vi "TurnDistance.vi"(7 "Timeout":dbl, 8 "Error In":errorcluster, 9 "Initation?":bool, 10 "MaxSpeed":dbl, 11 "Degrees":dbl) -> (0 "Error Out":errorcluster, 2 "Succesful":bool, 3 "Finished":bool)   [LabVIEW 2020]
uses:
  <vilib>/Utility/semaphor.llb/Obtain Semaphore Reference.vi
  <vilib>/Rock Robotics/WPI/ThirdParty/JAS_Junk/TrajLib/Timer_Reset.vi
  DriveGlobals.vi
  <vilib>/Rock Robotics/WPI/ThirdParty/JAS_Junk/TrajLib/Trajectory_Library.lvlib
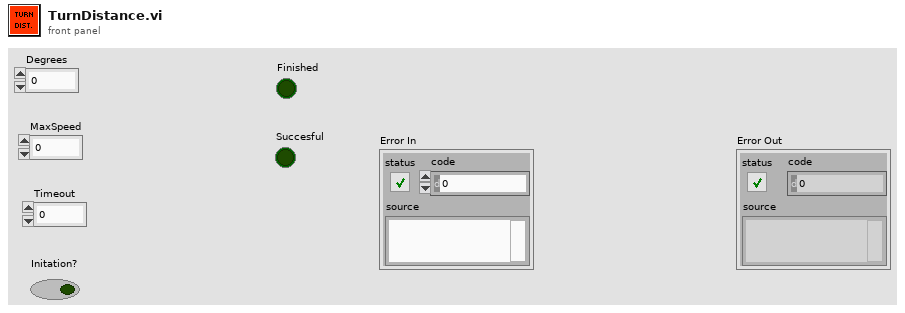
[diagram p1: front panel]
types:
  T1 = typedef "Trajectory_Library.lvlib/TIMER.ctl" = cluster{"StartTime":dbl, "Accumulated TIme":dbl, "Running":bool, "semaphore":T2}
  T2 = typedef "Semaphore RefNum" = refnum<k1>
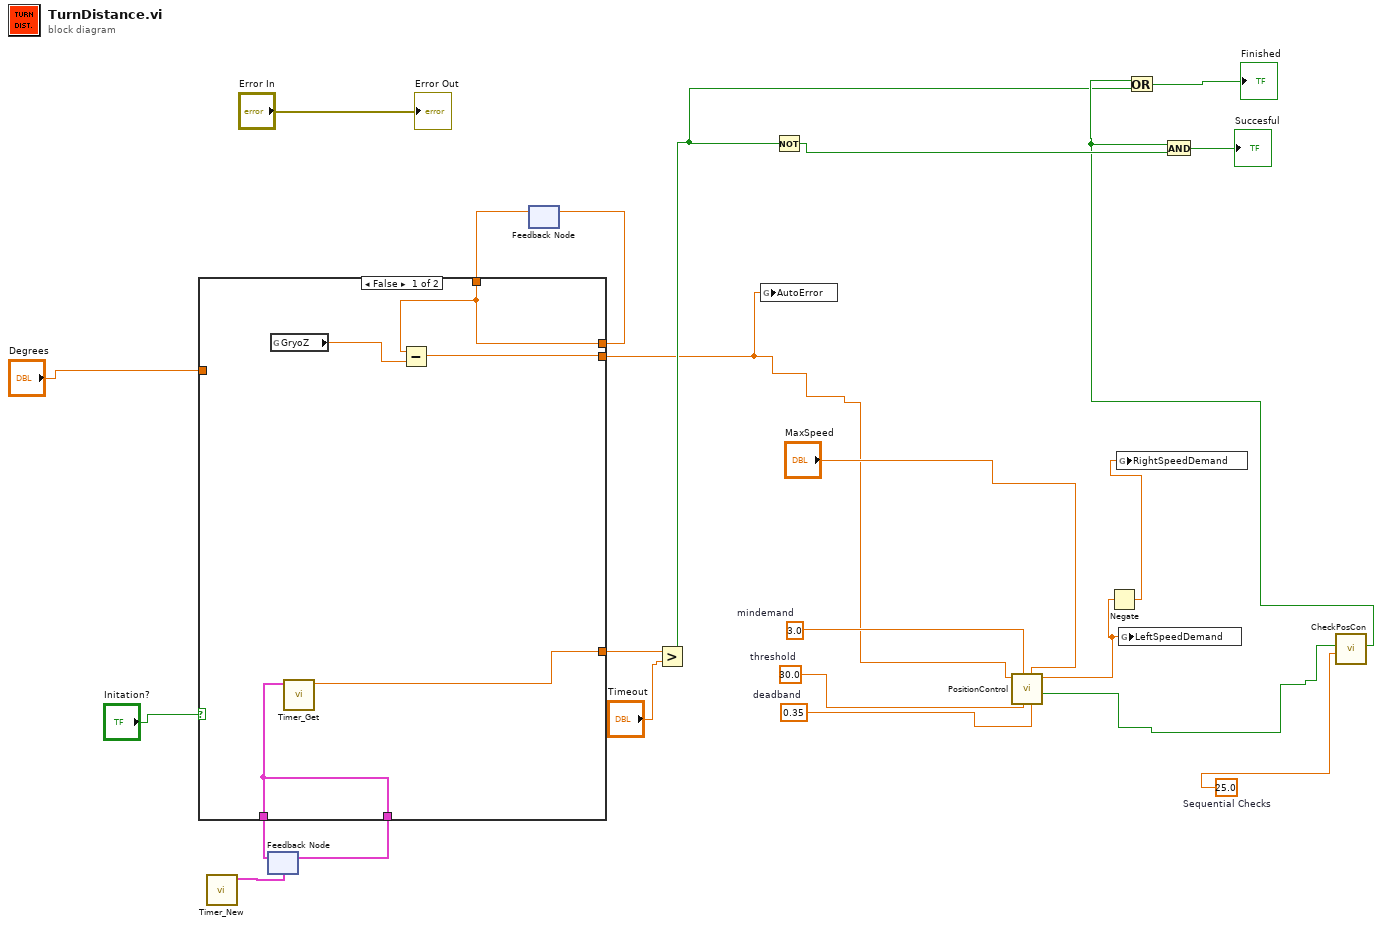
[diagram p0: block diagram]
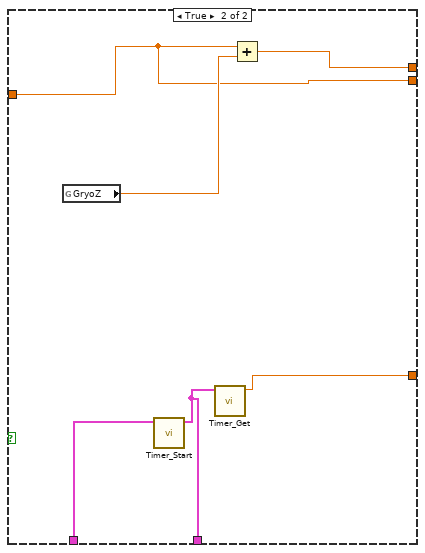
[diagram p2: hidden frame]
diagram:
  w8 = 25.0  # Sequential Checks
  w11 = 0.35  # deadband
  w10 = 30.0  # threshold
  w9 = 3.0  # mindemand
  n1 = call <vilib>:"Timer_New.vi"() -> ("TIMER"=w13:T1)  [unwired: 11 in]
  n2 = feedback #1(w13) -> (w22:T1)
  n3 = feedback #2() -> (w18:dbl)  [unwired: 1 in]
  n4 = case shown="False" "Initation?" {
    tunnel: w22 -> [w25 w31]
    tunnel: "Degrees" -> [_ w32]
    tunnel: w18 -> [w29 _]
    tunnel: [w29 w34] -> w19
    tunnel: [w27 w33] -> w14
    tunnel: [w26 w32] -> w1
    tunnel: [w25 w30] -> w12
    frame False {
      n5 = global read "DriveGlobals.vi" "GryoZ"() -> (w28:dbl)
      n6 = call <vilib>:"Timer_Get.vi"("TIMER"=w25) -> ("CurrentTImer"=w27:dbl)  [unwired: 10 in]
      n7 = Subtract(x=w29, y=w28) -> (x-y=w26:dbl)
    }
    frame True {
      n8 = global read "DriveGlobals.vi" "GryoZ"() -> (w35:dbl)
      n9 = call <vilib>:"Timer_Start.vi"("in Timer"=w31) -> ("out Timer"=w30:T1)  [unwired: 10 in]
      n10 = call <vilib>:"Timer_Get.vi"("TIMER"=w30) -> ("CurrentTImer"=w33:dbl)  [unwired: 10 in]
      n11 = Add(x=w32, y=w35) -> (x+y=w34:dbl)
    }
  }
  n12 = feedback-in #1(w12) -> ()
  n13 = feedback-in #2(w19) -> ()
  n14 = Greater?(x=w14, y="Timeout") -> (0:w2:bool)
  n15 = global write "DriveGlobals.vi" "AutoError"(w1) -> ()
  n16 = Not(x=w2) -> (.not. x?=w16:bool)
  n17 = call "PositionControl.vi"("deadband"=w11, "maxdemand"="MaxSpeed", "threshold"=w10, "mindemand"=w9, "Error"=w1) -> ("on target"=w5:bool, "output variable"=w4:dbl)  [unwired: 5 in]
  n18 = Negate(x=w4) -> (-x=w3:dbl)
  n19 = global write "DriveGlobals.vi" "RightSpeedDemand"(w3) -> ()
  n20 = global write "DriveGlobals.vi" "LeftSpeedDemand"(w4) -> ()
  n21 = call "CheckPosCon.vi"("Sequential Checks"=w8, "WasRight"=w5) -> ("We made It"=w7:bool)  [unwired: 9 in]
  n22 = Or(x=w7, y=w2) -> (x .or. y?=→"Finished":bool)
  n23 = And(x=w7, y=w16) -> (x .and. y?=→"Succesful":bool)
  "Error Out" <- "Error In"
